vi "WaveformChart.vi"() -> ()   [LabVIEW 2012]
panel:
  out "Waveform Chart":dbl(graph)
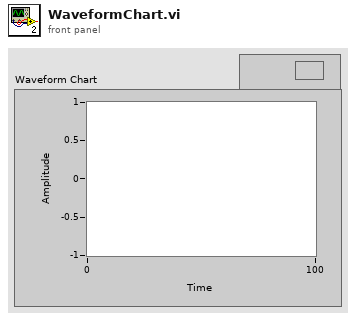
[diagram p1: front panel]
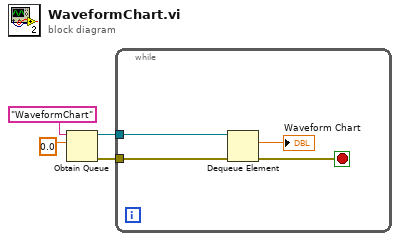
[diagram p0: block diagram]
diagram:
  n1 = Obtain Queue(name (unnamed)="WaveformChart", element data type=0.0 ("Waveform Chart")) -> (queue out=w1:refnum<queue>, error out=w4:errorcluster)  [unwired: 3 in, 1 out]
  n2 = while {
    tunnel: w4 -> [w8]
    tunnel: w1 -> [w7]
    stop <- w6 stop-if-true
    n3 = Dequeue Element(queue=w7, error in (no error)=w8) -> (element=→"Waveform Chart":dbl, error out=w6:errorcluster)  [unwired: 1 in, 2 out]
  }
